vi "GPS.vi"(9 "GPS In":refnum<visa-resource-name>) -> (0 "Robot Position":cluster{"Longitude":i32, "Latitude":i32} {"Latitude" format="%.7f"; "Longitude" format="%.7f"}, 3 "GPS out":refnum<visa-resource-name>)   [LabVIEW 2011]
doc: "This example shows how to acquire GPS data from a u-blox 5 GPS device with KickStart."
uses:
  <instrlib>/u-blox 5 Series/u-blox 5 Series.lvlib
panel:
  in  "Reset Before Reading (False)":bool
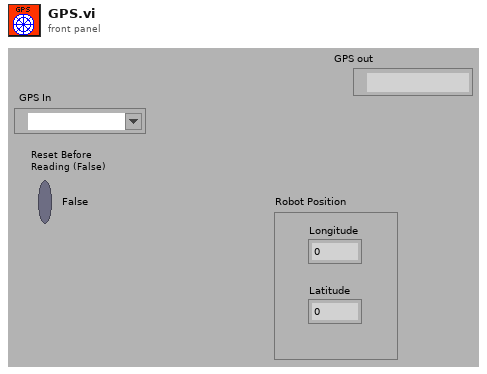
[diagram p1: front panel]
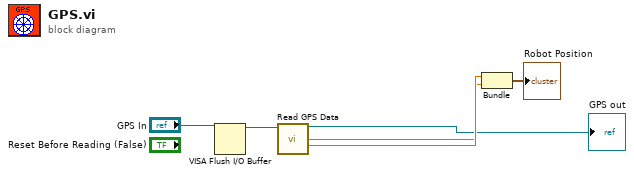
[diagram p0: block diagram]
diagram:
  n1 = VISA Flush I/O Buffer(VISA resource name="GPS In") -> (VISA resource name out=w1:refnum<visa-resource-name>)  [unwired: 2 in, 1 out]
  n2 = call <instrlib>:"Read GPS Data.vi"("VISA resource name"=w1) -> ("VISA resource name out"=→"GPS out":refnum<visa-resource-name>, "Latitude (°)"=w5:dbl, "Longitude (°)"=w6:dbl)  [unwired: 7 in, 5 out]
  n3 = Bundle("Longitude (°)"=w6, "Latitude (°)"=w5) -> (→"Robot Position":cluster{"Longitude (°)":dbl, "Latitude (°)":dbl})  [unwired: 1 in]
